vi "Convert Read ERD List to Message (Rev 2 API).vi"(0 "GEA Inputs":T2 {"Destination" format="%.0x"; "Source" format="%.0x"}, 7 "ERD Read Data In":T1 {"ERD Number" format="%.0x"}, 11 "Error In":errorcluster) -> (4 "GEA Message":T3 {"Command" format="%02x"; "Destination" format="%02x"; "Source" format="%02x"}, 6 "Request ID":string, 15 "Error Out":errorcluster)   [LabVIEW 2023, in "GEA2_Toolkit.lvlib"]
doc: "This vi uses the Source / Destination from the GEA input and the ERD list to format a single GEA2 message to read the list of ERDs."
uses:
  library/GEA2_Toolkit.lvlib
  type defs/Data In.ctl
  type defs/Source_Destination.ctl
  type defs/ERD Read Data In.ctl
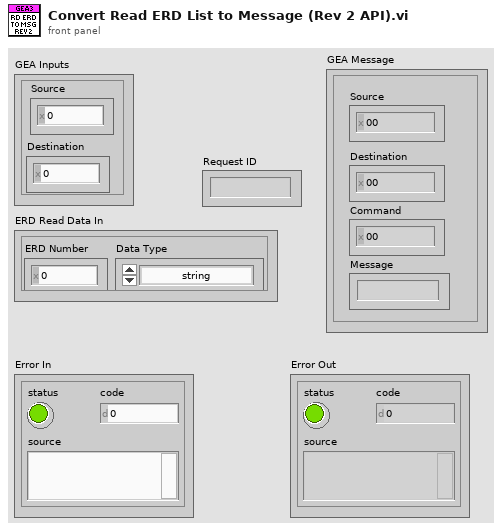
[diagram p1: front panel]
types:
  T1 = typedef "ERD Read Data In.ctl" = cluster{"ERD Number":u16, "Data Type":enum16{"string", "boolean", "uint8_t", "uint16_t", "uint32_t", "uint64_t", "int8_t", "int16_t", "int32_t", "int64_t"}}
  T2 = typedef "Source_Destination.ctl" = cluster{"Source":u8, "Destination":u8}
  T3 = typedef "Data In.ctl" = cluster{"Source":u8, "Destination":u8, "Command":u8, "Message":string}
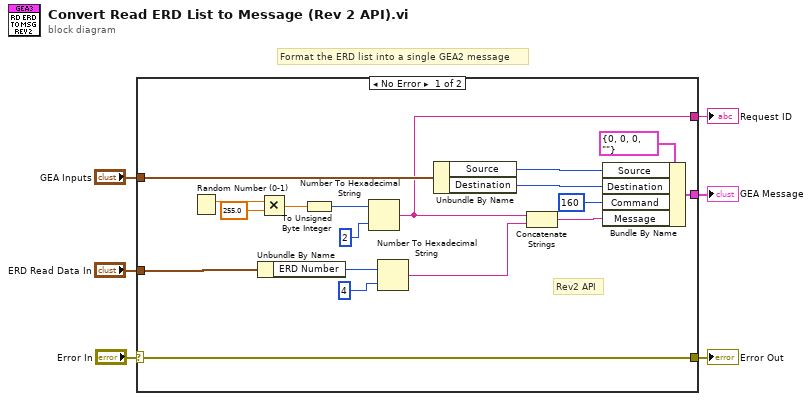
[diagram p0: block diagram]
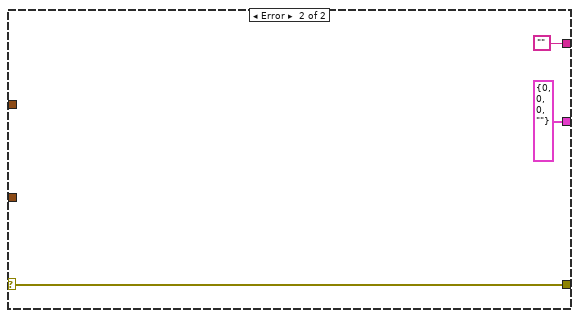
[diagram p2: hidden frame]
diagram:
  # "Format the ERD list into a single GEA2 message"
  n1 = case shown="No Error" "Error In" {
    selector: "Error In" -> [w16 w26]
    tunnel: "ERD Read Data In" -> [w7 _]
    tunnel: "GEA Inputs" -> [w22 _]
    tunnel: [w17 T3 {"Source"=0, "Destination"=0, "Command"=0, "Message"=""} ("GEA Message")] -> w5
    tunnel: [w16 w26] -> w3
    tunnel: [w11 ""] -> w2
    frame No Error {
      # "Rev2 API"
      n2 = Random Number (0-1)() -> (number: 0 to 1=w15:dbl)
      n3 = Unbundle By Name(w7) -> ("ERD Number"=w9:u16)
      n4 = Multiply(x=w15, y=255.0) -> (x*y=w13:dbl)
      n5 = To Unsigned Byte Integer(number=w13) -> (unsigned 8bit integer=w12:u8)
      n6 = Number To Hexadecimal String(1:i16 2 ("width (-)"), 2:w12) -> (0:w11:string)
      n7 = Number To Hexadecimal String(1:i16 4 ("width (-)"), 2:w9) -> (0:w8:string)
      n8 = Unbundle By Name(w22) -> ("Source"=w21:u8, "Destination"=w20:u8)
      n9 = Concatenate Strings(w11, w8) -> (w18:string)
      n10 = Bundle By Name(cluster=T3 {"Source"=0, "Destination"=0, "Command"=0, "Message"=""} ("GEA Message"), "Source"=w21, "Destination"=w20, "Command"=u8 160, "Message"=w18) -> (w17:T3)
    }
    frame Error {
    }
  }
  "GEA Message" <- w5
  "Error Out" <- w3
  "Request ID" <- w2
